vi "Photo Get Illuminance.vi"(8 "error in (no error)":errorcluster, 10 "a_CIEResolution":u8, 11 "a_data":dbl[](array[numeric])) -> (0 "error out":errorcluster, 1 "a_Lux out":dbl, 2 "function return":i16, 3 "a_data out":dbl[](array[numeric]))   [LabVIEW 2013, in "AvaSpec.lvlib" / "AVSirrad_support.lvlib" / "AVSirrad.lvlib"]
doc: "DLL_API short int __stdcall Photo_GetIlluminance\n(\n DataType *a_data,\n unsigned char a_CIEResolution,\n double *a_Lux\n\n);"
uses:
  AVSirrad.lvlib
  AVSIRRAD/Examples/Labview/build/AVSirrad.dll
panel:
  in  "a_Lux":dbl
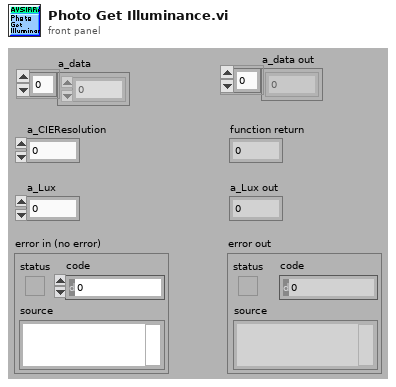
[diagram p1: front panel]
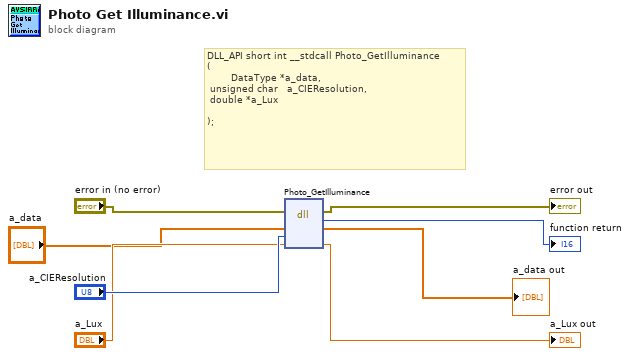
[diagram p0: block diagram]
diagram:
  # "DLL_API short int __stdcall Photo_GetIlluminance\n(\n        DataType *a_data,\n\tunsigned char   a_CIEResolution,\n\tdouble *a_Lux\n\n);"
  n1 = dll-call lib="C:/AVSIRRAD/Examples/Labview/build/AVSirrad.*" fn="Photo_GetIlluminance"(error in="error in (no error)", "a_data"="a_data", "a_CIEResolution"="a_CIEResolution", "a_Lux"="a_Lux") -> (error out=→"error out":errorcluster, "return type"=→"function return":i16, "a_data"=→"a_data out":dbl[], "a_Lux"=→"a_Lux out":dbl)  [unwired: 3 in, 1 out]
